vi "Name Value Get User Input.vi"(7 "Dialog Message":string) -> (4 "User Input":string, 15 "Canceled?":bool)   [LabVIEW 2020]
uses:
  <vilib>/Utility/miscctls.llb/LVPointTypeDef.ctl
  <vilib>/Utility/error.llb/whitespace.ctl
panel:
  in  "Get User Input":string caption="Add Buffer Type:"
  in  "Cancel":bool
  in  "Done":bool
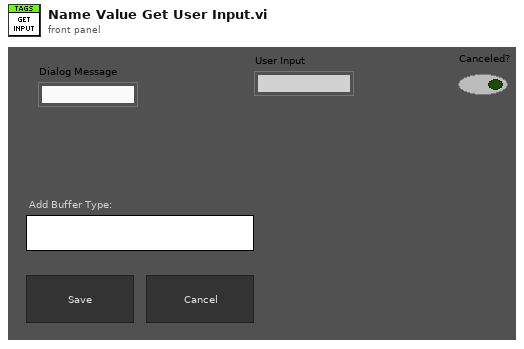
[diagram p1: front panel]
types:
  T1 = enum16{"Always On", "Always Off", "Off While Running"}
  T2 = typedef "LVPointTypeDef.ctl" = cluster{"Horizontal":i16, "Vertical":i16}
  T3 = typedef "LVRectTypeDef.ctl" = cluster{"Left":i16, "Top":i16, "Right":i16, "Bottom":i16}
  T4 = typedef "LVBoundsTypeDef.ctl" = cluster{"Width":u32, "Height":u32}
  T5 = typedef "whitespace.ctl" = u16
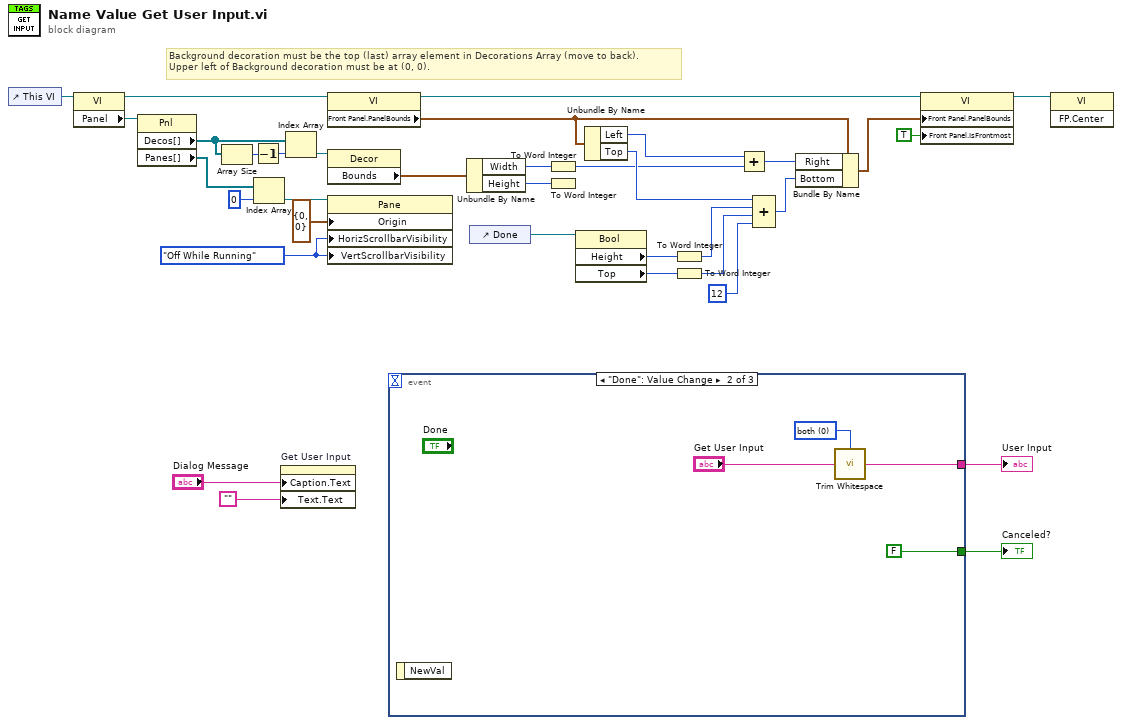
[diagram p0: block diagram]
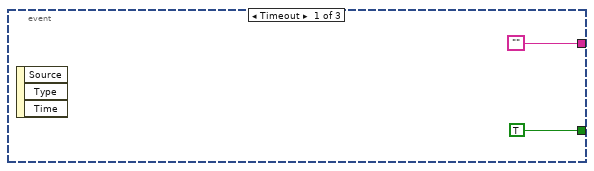
[diagram p2: hidden frame]
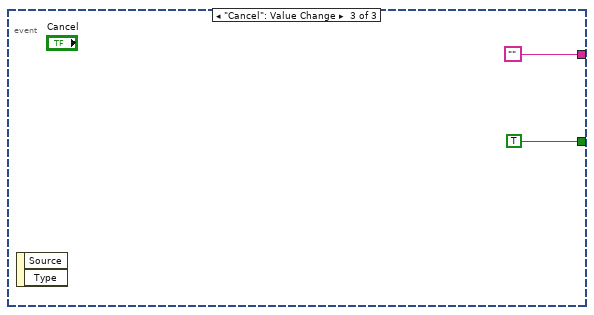
[diagram p3: hidden frame]
diagram:
  w18 = T1."Off While Running" ("Vertical Scrollbar Visibility")
  # "Background decoration must be the top (last) array element in Decorations Array (move to back).\nUpper left of Background decoration must be at (0, 0)."
  n1 = control-ref of="This VI"() -> (w10:refnum<vi>)
  n2 = property class="VI"(reference=w10) -> (reference out=w19:refnum<vi>, "Panel"=w11:refnum<vi>)  [unwired: 1 in, 1 out]
  n3 = property class="Pnl"(reference=w11) -> ("Decos[]"=w9:refnum<vi>[], "Panes[]"=w15:refnum<vi>[])  [unwired: 1 in, 2 out]
  n4 = Array Size(array=w9) -> (size(s)=w7:i32)
  n5 = Decrement(x=w7) -> (x-1=w8:i32)
  n6 = Index Array(array=w15, index=0) -> (element=w14:refnum<vi>)
  n7 = property on="Get User Input" class="Str"("Caption.Text"="Dialog Message", "Text.Text"="") -> ()  [unwired: 2 in, 2 out]
  n8 = Index Array(array=w9, index=w8) -> (element=w17:refnum<vi>)
  n9 = property class="VI"(reference=w19) -> (reference out=w21:refnum<vi>, "Front Panel.PanelBounds"=w22:T3)  [unwired: 1 in, 1 out]
  n10 = property class="Decor"(reference=w17) -> ("Bounds"=w20:T4)  [unwired: 1 in, 2 out]
  n11 = property class="Pane"(reference=w14, "Origin"=T2 {"Horizontal"=0, "Vertical"=0}, "HorizScrollbarVisibility"=w18, "VertScrollbarVisibility"=w18) -> ()  [unwired: 1 in, 2 out]
  n12 = event shown="[1] \"Done\": Value Change" {
    selector: _ -> [_ _ _]
    dyn-events: _ -> [_ _ _]
    timeout: _ -> [_ _ _]
    tunnel: ["" w39 ""] -> w3
    tunnel: [TRUE FALSE TRUE] -> w2
    event Timeout {
      n13 = event-data() -> ()  [unwired: 1 in, 3 out]
    }
    event "Done": Value Change {
      w38 = T5 0 items=["both", "start of string", "end of string"] ("location (both)")
      n14 = event-data() -> ()  [unwired: 1 in, 1 out]
      n15 = call <vilib>:"Trim Whitespace.vi"("string"="Get User Input", "location (both)"=w38) -> ("trimmed string"=w39:string)
    }
    event "Cancel": Value Change {
      n16 = event-data() -> ()  [unwired: 1 in, 2 out]
    }
  }
  "Canceled?" <- w2
  "User Input" <- w3
  n17 = Unbundle By Name(w20) -> ("Width"=w25:u32, "Height"=w28:u32)
  n18 = control-ref of="Done"() -> (w12:refnum<vi>)
  n19 = To Word Integer(number=w25) -> (16bit integer=w27:i16)
  n20 = To Word Integer(number=w28) -> ()  [unwired: 1 out]
  n21 = property class="Bool"(reference=w12) -> ("Height"=w30:u32, "Top"=w31:i32)  [unwired: 1 in, 2 out]
  n22 = Unbundle By Name(w22) -> ("Left"=w24:i16, "Top"=w35:i16)
  n23 = To Word Integer(number=w30) -> (16bit integer=w33:i16)
  n24 = To Word Integer(number=w31) -> (16bit integer=w34:i16)
  n25 = Add(x=w24, y=w27) -> (x+y=w26:i16)
  n26 = Compound Arithmetic op=ADD(w35, w33, w34, i16 12 ("y")) -> (w29:i16)
  n27 = Bundle By Name(cluster=w22, "Right"=w26, "Bottom"=w29) -> (w23:T3)
  n28 = property class="VI"(reference=w21, "Front Panel.PanelBounds"=w23, "Front Panel.IsFrontmost"=TRUE ("Front Panel Window:Is Frontmost")) -> (reference out=w5:refnum<vi>)  [unwired: 1 in, 1 out]
  n29 = invoke class="VI" method="FP.Center"(reference=w5) -> ()  [unwired: 2 in, 3 out]
